vi "Lock focus.vi"(8 "error in":errorcluster, 11 "VISA resource in":refnum<visa-resource-name>) -> (0 "error out":errorcluster, 3 "VISA resource out":refnum<visa-resource-name>)   [LabVIEW 2018]
panel:
  out "Status before lock attempt":string
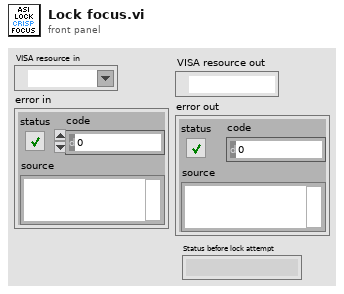
[diagram p1: front panel]
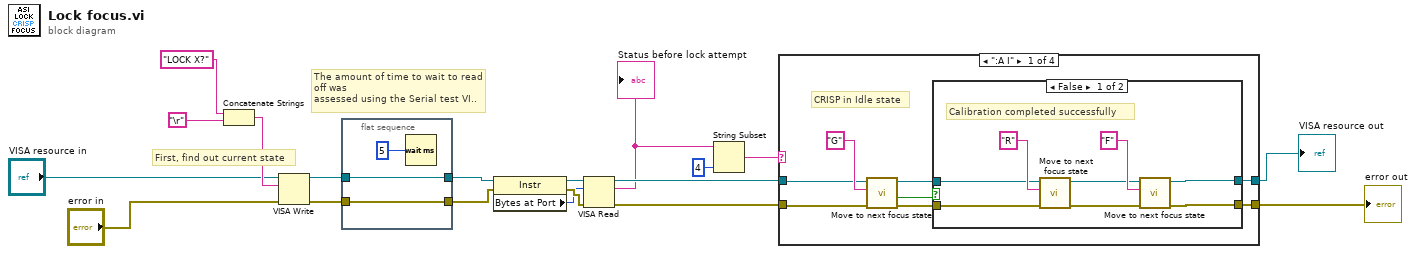
[diagram p0: block diagram]
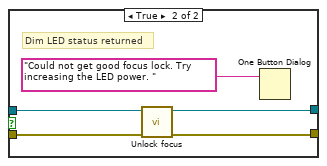
[diagram p2: hidden frame]
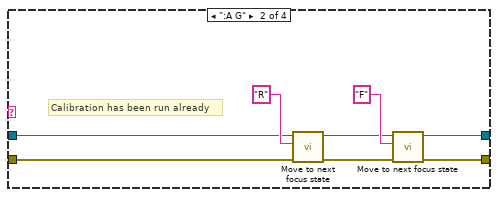
[diagram p3: hidden frame]
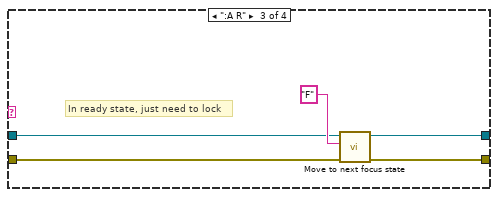
[diagram p4: hidden frame]
diagram:
  # "The amount of time to wait to read off was \nassessed using the Serial test VI.."
  # "First, find out current state"
  n1 = Concatenate Strings("LOCK X?" ("write buffer"), "\r") -> (w9:string)
  n2 = VISA Write(VISA resource name="VISA resource in", write buffer=w9, error in (no error)="error in") -> (VISA resource name out=w15:refnum<visa-resource-name>, error out=w14:errorcluster)  [unwired: 1 out]
  n3 = flat-sequence {
    tunnel: [w22] -> w12
    tunnel: w15 -> [w22]
    tunnel: [w20] -> w13
    tunnel: w14 -> [w20]
    frame #0 {
      n4 = Wait (ms)(milliseconds to wait=u32 5) -> ()  [unwired: 1 out]
    }
  }
  n5 = property class="Instr"(reference=w12, error in=w13) -> (reference out=w16:refnum<visa-resource-name>, error out=w18:errorcluster, "Bytes at Port"=w17:u32)
  n6 = VISA Read(VISA resource name=w16, byte count=w17, error in (no error)=w18) -> (VISA resource name out=w10:refnum<visa-resource-name>, read buffer=w1:string, error out=w11:errorcluster)  [unwired: 1 out]
  "Status before lock attempt" <- w1
  n7 = String Subset(string=w1, length (rest)=4 ("length (rest)")) -> (substring=w3:string)  [unwired: 1 in]
  n8 = case shown="\":A I\"" w3 {
    tunnel: w11 -> [w28 w46 w54 w57]
    tunnel: w10 -> [w29 w47 w55 w58]
    tunnel: [w24 w44 w52 w57] -> w4
    tunnel: [w25 w45 w53 w58] -> w5
    frame ":A I" {
      # "CRISP in Idle state"
      n9 = call "Move to next focus state.vi"("error in"=w28, "Next state indicator"="G", "VISA resource in"=w29) -> ("error out"=w27:errorcluster, "LED TOO DIM?"=w23:bool, "VISA resource out"=w26:refnum<visa-resource-name>)  [unwired: 6 in]
      n10 = case shown="False" w23 {
        tunnel: w27 -> [w37 w40]
        tunnel: w26 -> [w36 w43]
        tunnel: [w32 w42] -> w25
        tunnel: [w31 w41] -> w24
        frame False {
          # "Calibration completed successfully"
          n11 = call "Move to next focus state.vi"("error in"=w37, "Next state indicator"="R", "VISA resource in"=w36) -> ("error out"=w33:errorcluster, "VISA resource out"=w34:refnum<visa-resource-name>)  [unwired: 6 in, 1 out]
          n12 = call "Move to next focus state.vi"("error in"=w33, "Next state indicator"="F", "VISA resource in"=w34) -> ("error out"=w31:errorcluster, "VISA resource out"=w32:refnum<visa-resource-name>)  [unwired: 6 in, 1 out]
        }
        frame True {
          # "Dim LED status returned"
          n13 = call "Unlock focus.vi"("error in"=w40, "VISA resource in"=w43) -> ("error out"=w41:errorcluster, "VISA resource out"=w42:refnum<visa-resource-name>)  [unwired: 8 in]
          n14 = One Button Dialog(message="Could not get good focus lock. Try increasing the LED power. ") -> ()  [unwired: 1 in, 1 out]
        }
      }
    }
    frame ":A G" {
      # "Calibration has been run already"
      n15 = call "Move to next focus state.vi"("error in"=w46, "Next state indicator"="R", "VISA resource in"=w47) -> ("error out"=w48:errorcluster, "VISA resource out"=w49:refnum<visa-resource-name>)  [unwired: 6 in, 1 out]
      n16 = call "Move to next focus state.vi"("error in"=w48, "Next state indicator"="F", "VISA resource in"=w49) -> ("error out"=w44:errorcluster, "VISA resource out"=w45:refnum<visa-resource-name>)  [unwired: 6 in, 1 out]
    }
    frame ":A R" {
      # "In ready state, just need to lock"
      n17 = call "Move to next focus state.vi"("error in"=w54, "Next state indicator"="F", "VISA resource in"=w55) -> ("error out"=w52:errorcluster, "VISA resource out"=w53:refnum<visa-resource-name>)  [unwired: 6 in, 1 out]
    }
    frame ":A F", Default {
      # "Already in focussed state"
    }
  }
  "VISA resource out" <- w5
  "error out" <- w4
